vi "LIN Frame 2 Data.vi"(2 "Frame":string) -> (1 "Array OUT":u8[](array[numeric]), 4 "Element":string[](array[string]), 5 "Error?":bool, 6 "Get Key?":bool, 7 "MulFrame":bool, 8 "Finish?":bool)   [LabVIEW 2018]
uses:
  <vilib>/regexp/Match Regular Expression.xnode
panel:
  out "Numeric":i32
  out "offset past match":i32
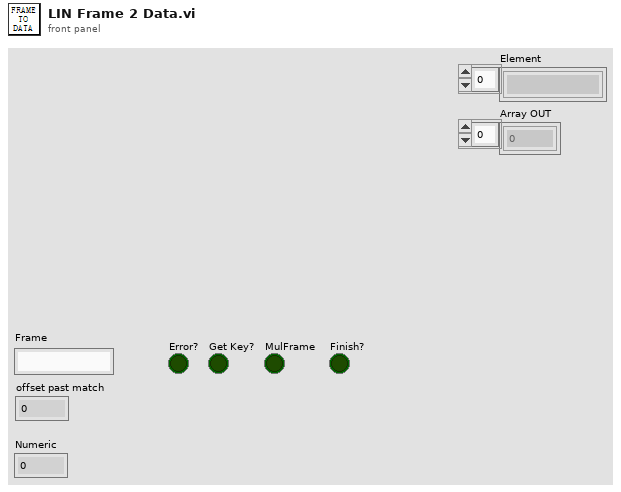
[diagram p1: front panel]
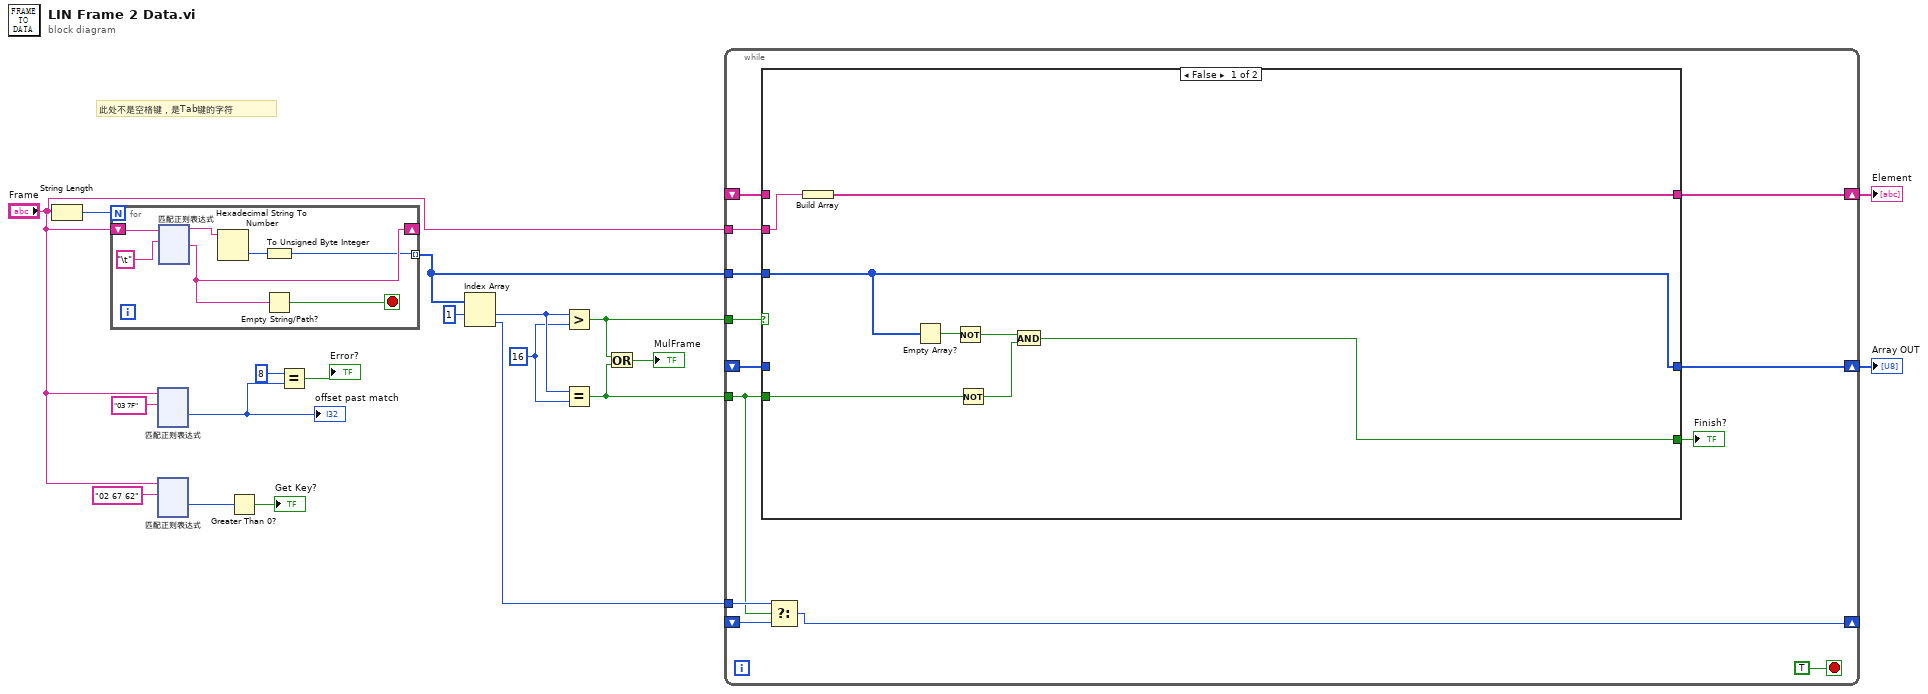
[diagram p0: block diagram]
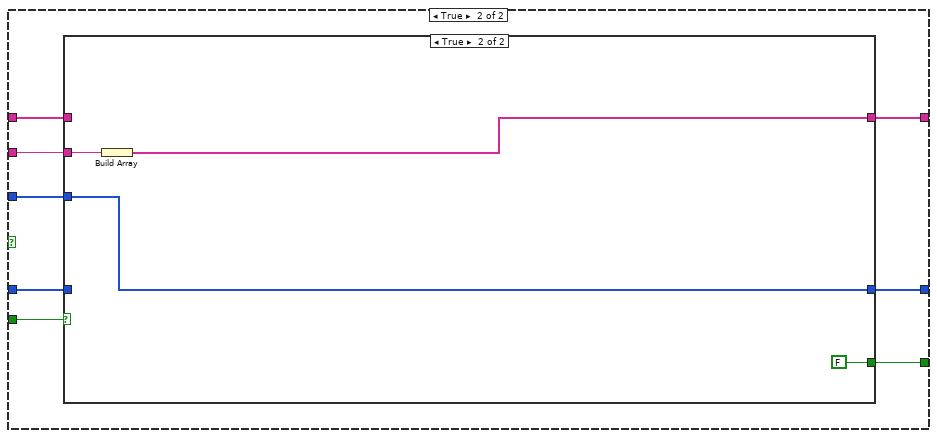
[diagram p2: hidden frame]
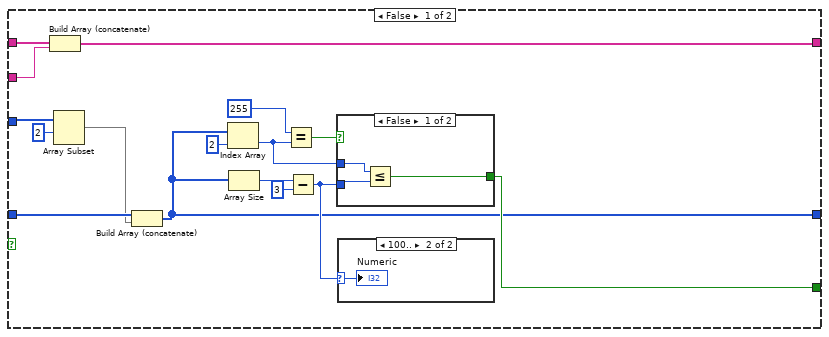
[diagram p3: hidden frame]
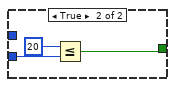
[diagram p5: hidden frame]
diagram:
  w9 = u8 16 ("y")
  # "此处不是空格键，是Tab键的字符"
  n1 = String Length(string="Frame") -> (length=w19:i32)
  n2 = for {
    N: w19 -> [_]
    shift-right: [w23] -> _
    shift-left: "Frame" -> [w26]
    tunnel: [w22] -> w8 mode=indexing
    stop <- w24 stop-if-true
    n3 = xnode "匹配正则表达式"("输入字符串"=w26, "正则表达式"="\t") -> ("匹配之前"=w21:string, "匹配之后"=w23:string)  [unwired: 4 in, 3 out]
    n4 = Hexadecimal String To Number(string=w21) -> (number=w25:u32)  [unwired: 2 in, 1 out]
    n5 = To Unsigned Byte Integer(number=w25) -> (unsigned 8bit integer=w22:u8)
    n6 = Empty String/Path?(string/path=w23) -> (empty?=w24:bool)
  }
  n7 = xnode "匹配正则表达式"("输入字符串"="Frame", "正则表达式"="03 7F") -> ("匹配后偏移量"=w16:i32)  [unwired: 4 in, 4 out]
  "offset past match" <- w16
  n8 = xnode "匹配正则表达式"("输入字符串"="Frame", "正则表达式"="02 67 62") -> ("匹配后偏移量"=w13:i32)  [unwired: 4 in, 4 out]
  n9 = Greater Than 0?(x=w13) -> (x > 0?=→"Get Key?":bool)
  n10 = Equal?(x=8, y=w16) -> (x = y?=→"Error?":bool)
  n11 = Index Array(array=w8, index #1=1 ("索引")) -> (element #1=w10:u8, element #2=w7:u8)  [unwired: 1 in]
  n12 = Greater?(x=w10, y=w9) -> (0:w6:bool)
  n13 = Equal?(x=w10, y=w9) -> (x = y?=w5:bool)
  n14 = Or(x=w6, y=w5) -> (x .or. y?=→"MulFrame":bool)
  n15 = while {
    tunnel: w6 -> [w153]
    tunnel: w5 -> [w142]
    tunnel: "Frame" -> [w152]
    shift-right: [w151] -> w3
    shift-left: _ -> [w150]
    tunnel: w8 -> [w149]
    shift-right: [w148] -> w2
    shift-left: _ -> [w147]
    shift-right: [w141] -> _
    shift-left: _ -> [w143]
    tunnel: w7 -> [w144]
    stop <- TRUE stop-if-true
    n16 = case shown="False" w153 {
      tunnel: w142 -> [w157 w169]
      tunnel: w152 -> [w161 w168]
      tunnel: [w160 w167] -> w151
      tunnel: w150 -> [_ w166]
      tunnel: w149 -> [w154 w165]
      tunnel: [w154 w164] -> w148
      tunnel: w147 -> [_ w163]
      tunnel: [w155 w162] -> w145
      frame False {
        n17 = Build Array(w161) -> (w160:string[])
        n18 = Empty Array?(array=w154) -> (empty?=w159:bool)
        n19 = Not(x=w159) -> (.not. x?=w158:bool)
        n20 = Not(x=w157) -> (.not. x?=w156:bool)
        n21 = And(x=w158, y=w156) -> (x .and. y?=w155:bool)
      }
      frame True {
        n22 = case shown="True" w169 {
          tunnel: w168 -> [w185 w196]
          tunnel: [w183 w195] -> w167
          tunnel: w166 -> [w184 _]
          tunnel: w165 -> [w182 w194]
          tunnel: [w170 w194] -> w164
          tunnel: w163 -> [w180 _]
          tunnel: [w172 FALSE] -> w162
          frame False {
            n23 = Build Array (concatenate)(w184, w185) -> (w183:string[])
            n24 = Array Subset(array=w182, index=2 ("索引")) -> (w179:u8[])  [unwired: 1 in]
            n25 = Build Array (concatenate)(w180, w179) -> (w170:u8[])
            n26 = Index Array(array=w170, index=2 ("索引 (行)")) -> (element=w175:u8)
            n27 = Array Size(array=w170) -> (size(s)=w174:i32)
            n28 = Equal?(x=u8 255 ("索引 (行)"), y=w175) -> (x = y?=w176:bool)
            n29 = Subtract(x=w174, y=3) -> (x-y=w171:i32)
            n30 = case shown="False" w176 {
              tunnel: w175 -> [w189 _]
              tunnel: w171 -> [w188 w192]
              tunnel: [w187 w190] -> w172
              frame False {
                n31 = Less Or Equal?(x=w189, y=w188) -> (x <= y?=w187:bool)
              }
              frame True {
                n32 = Less Or Equal?(x=20, y=w192) -> (x <= y?=w190:bool)
              }
            }
            n33 = case shown="100.." w171 {
              selector: w171 -> [_ w186]
              frame Default {
              }
              frame 100.. {
                "Numeric" <- w186
              }
            }
          }
          frame True {
            n34 = Build Array(w196) -> (w195:string[])
          }
        }
      }
    }
    "Finish?" <- w145
    n35 = Select(t=w144, s=w142, f=w143) -> (s? t:f=w141:u8)
  }
  "Element" <- w3
  "Array OUT" <- w2
